vi "Allocate Memory.vi"(3 "Error In":errorcluster, 5 "Type Descriptor":string) -> (0 "Error Out":errorcluster, 1 "Data":string, 2 "dup Type Descriptor":string)   [LabVIEW 2014, in "CS++DIM.lvlib" / "DIMConnection.lvclass"]
doc: "Allocate memory for DIM service to publish."
uses:
  DIMConnection.lvclass
  CSPP_Core/Libraries/Utilities/CS++Utilities.lvlib
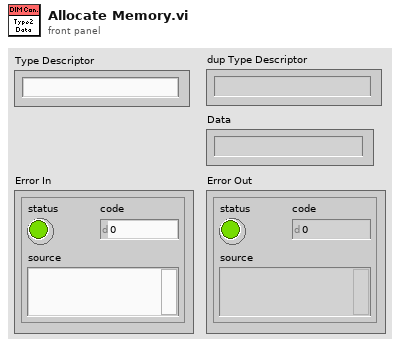
[diagram p1: front panel]
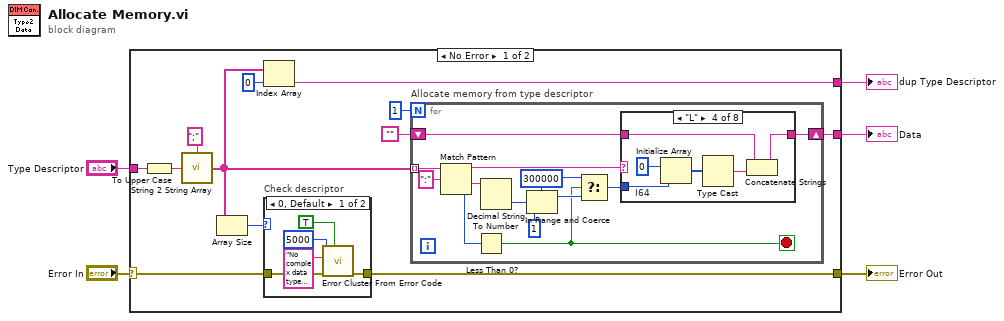
[diagram p0: block diagram]
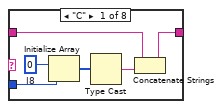
[diagram p3: hidden frame]
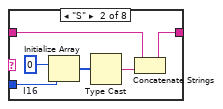
[diagram p4: hidden frame]
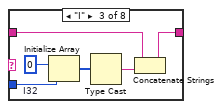
[diagram p5: hidden frame]
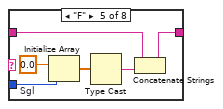
[diagram p6: hidden frame]
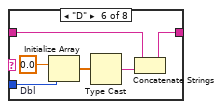
[diagram p7: hidden frame]
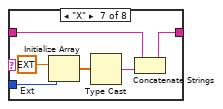
[diagram p8: hidden frame]
diagram:
  n1 = case shown="No Error" "Error In" {
    selector: "Error In" -> [w6 w81]
    tunnel: "Type Descriptor" -> [w16 w80]
    tunnel: [w14 _] -> w4
    tunnel: [w9 w80] -> w3
    tunnel: [w7 w81] -> w2
    frame No Error {
      n2 = To Upper Case(1:w16) -> (0:w10:string)
      n3 = call "String 2 String Array.vi"("String"=w10, "Delimiter (\",\")"=";" ("Delimiter (\",\")")) -> ("Substrings"=w11:string[])
      n4 = Array Size(array=w11) -> (size(s)=w13:i32)
      n5 = Index Array(array=w11, index=0) -> (element=w9:string)
      n6 = case "Check descriptor" shown="0, Default" w13 {
        tunnel: w6 -> [w22 w23]
        tunnel: [w21 w23] -> w7
        frame 0, Default {
          n7 = call <vilib>:"Error Cluster From Error Code.vi"("show call chain? (False)"=TRUE, "error in (no error)"=w22, "error message (\"\")"="No complex data types support for now." ("error message (\"\")"), "error code (0)"=5000) -> ("error out"=w21:errorcluster)  [unwired: 5 in]
        }
        frame 1 {
        }
      }
      n8 = for "Allocate memory from type descriptor" {
        N: 1 -> [_]
        tunnel: w11 -> [w34] mode=indexing
        shift-right: [w36] -> w14
        shift-left: "" -> [w35]
        stop <- w24 stop-if-true
        w27 = 300000 ("upper limit")
        n9 = Match Pattern(string=w34, regular expression=":") -> (before substring=w33:string, after substring=w31:string, offset past match=w28:i32)  [unwired: 1 in, 1 out]
        n10 = Less Than 0?(x=w28) -> (x < 0?=w24:bool)
        n11 = Decimal String To Number(string=w31) -> (number=w29:i32)  [unwired: 2 in, 1 out]
        n12 = In Range and Coerce(upper limit=w27, x=w29, lower limit=1) -> (coerced(x)=w26:i32)  [unwired: 1 out]
        n13 = Select(t=w27, s=w24, f=w26) -> (s? t:f=w25:i32)
        n14 = case shown="\"L\"" w33 {
          tunnel: [w41 w47 w53 w59 w65 w71 w77 w79] -> w36
          tunnel: w35 -> [w42 w48 w54 w60 w66 w72 w78 w79]
          tunnel: w25 -> [w37 w43 w49 w55 w61 w67 w73 _]
          frame "C" {
            w39 = i8 0  # I8
            n15 = Initialize Array(w39, w37) -> (w38:i8[])
            n16 = Type Cast(x=w38) -> (*(type *) &x=w40:string)  [unwired: 1 in]
            n17 = Concatenate Strings(w42, w40) -> (w41:string)
          }
          frame "S" {
            w45 = i16 0  # I16
            n18 = Initialize Array(w45, w43) -> (w44:i16[])
            n19 = Type Cast(x=w44) -> (*(type *) &x=w46:string)  [unwired: 1 in]
            n20 = Concatenate Strings(w48, w46) -> (w47:string)
          }
          frame "I" {
            w51 = 0  # I32
            n21 = Initialize Array(w51, w49) -> (w50:i32[])
            n22 = Type Cast(x=w50) -> (*(type *) &x=w52:string)  [unwired: 1 in]
            n23 = Concatenate Strings(w54, w52) -> (w53:string)
          }
          frame "L" {
            w57 = i64 0  # I64
            n24 = Initialize Array(w57, w55) -> (w56:i64[])
            n25 = Type Cast(x=w56) -> (*(type *) &x=w58:string)  [unwired: 1 in]
            n26 = Concatenate Strings(w60, w58) -> (w59:string)
          }
          frame "F" {
            w63 = sgl 0.0  # Sgl
            n27 = Initialize Array(w63, w61) -> (w62:sgl[])
            n28 = Type Cast(x=w62) -> (*(type *) &x=w64:string)  [unwired: 1 in]
            n29 = Concatenate Strings(w66, w64) -> (w65:string)
          }
          frame "D" {
            w69 = 0.0  # Dbl
            n30 = Initialize Array(w69, w67) -> (w68:dbl[])
            n31 = Type Cast(x=w68) -> (*(type *) &x=w70:string)  [unwired: 1 in]
            n32 = Concatenate Strings(w72, w70) -> (w71:string)
          }
          frame "X" {
            w75 = ext 0.0  # Ext
            n33 = Initialize Array(w75, w73) -> (w74:ext[])
            n34 = Type Cast(x=w74) -> (*(type *) &x=w76:string)  [unwired: 1 in]
            n35 = Concatenate Strings(w78, w76) -> (w77:string)
          }
          frame Default {
          }
        }
      }
    }
    frame Error {
    }
  }
  "dup Type Descriptor" <- w3
  "Data" <- w4
  "Error Out" <- w2
